vi "Get Core.vi"(8 "Error In":errorcluster, 11 "WebView in":refnum<class "WebView.lvclass">) -> (0 "Error Out":errorcluster, 2 "Core":refnum<k24>, 3 "WebView out":refnum<class "WebView.lvclass">)   [LabVIEW 2024, in "WebView.lvclass"]
uses:
  WebView.lvclass
  <vilib>/sklein/WebView2/Libs/Microsoft.Web.WebView2.Core.dll
  WebView.lvclass/WebView.ctl
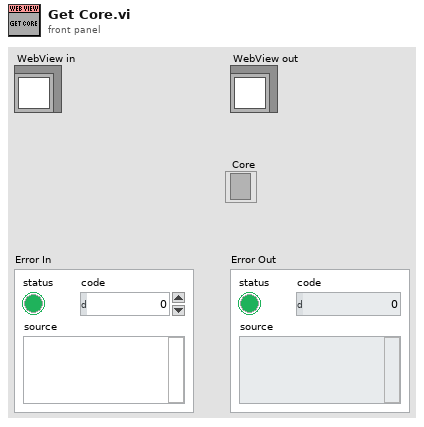
[diagram p1: front panel]
types:
  T1 = typedef "WebView.lvclass/Resources--cluster.ctl" = cluster{"WebView2 Control":refnum<k24>, "Webview2 Core":refnum<k24>, "event callback":refnum<k27>, "Environment":refnum<k24>}
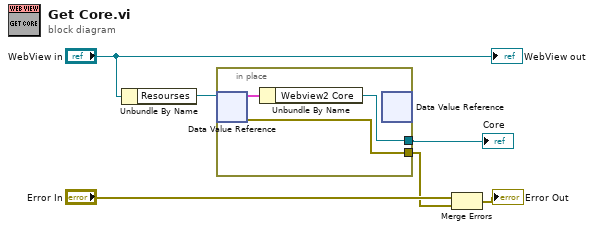
[diagram p0: block diagram]
diagram:
  n1 = Unbundle By Name("WebView in") -> ("Resourses"=w5:refnum<data-value>)
  n2 = in-place {
    in-place-border: [w8] -> w2
    in-place-border: [w7] -> w3
    n3 = in-place-dvr #1(w5) -> (w9:T1, w7:errorcluster)
    n4 = Unbundle By Name(w9) -> ("Webview2 Core"=w8:refnum<k24>)
    n5 = in-place-dvr #1() -> ()  [unwired: 1 in, 2 out]
  }
  "Core" <- w2
  n6 = Merge Errors("Error In", w3) -> (→"Error Out":errorcluster)
  "WebView out" <- "WebView in"
